vi "TP-PONDUL-INVERSE-PID.vi"() -> ()   [LabVIEW 2018]
uses:
  <vilib>/Instr/_visa.llb/VISA Configure Serial Port (Instr).vi
  <vilib>/addons/control/pid/pid.llb/PID (DBL).vi
  <vilib>/addons/control/pid/NI_PID_pid.lvlib
panel:
  in  "Tab Control":enum32{"Page 0", "Page 1", "Page 2"}(tab)
  out "Waveform Chart":dynamicdata(graph)
  in  "Consigne":dbl(knob) scale=-10.0..10.0
  out "Mesure":dbl(knob) scale=-50.0..50.0
  in  "stop":bool
  in  "VISA resource name":refnum<visa-resource-name>
  in  "PID gains":cluster{"P":dbl, "I":dbl, "D":dbl}={"P"=1.0, "I"=0.01, "D"=0.0} {"D" scale=0.0..28.0; "I" scale=0.0..0.0001; "P" scale=0.0..45.0}
  out "SPEED":dbl
  # "UNIVESITE SULTAN MOULAY SLIMANE\nFACULTE DES SCIENCES ET TECHNIQUES DE BENI MELLAL"
  # "Réalisé par : BANANE Mohamed\n               IDRRISI Hamza\n                      BELAISSAOUI ARBI\n                          TACHTIOUINE Hicham\n              CHAMIT Salim"
  # "Encadré par : Pr. KHAOUCH Zakaria"
  # "Placez tout \nd'abord le \npendule dans \nsa position d'equilibre \nverticale !"
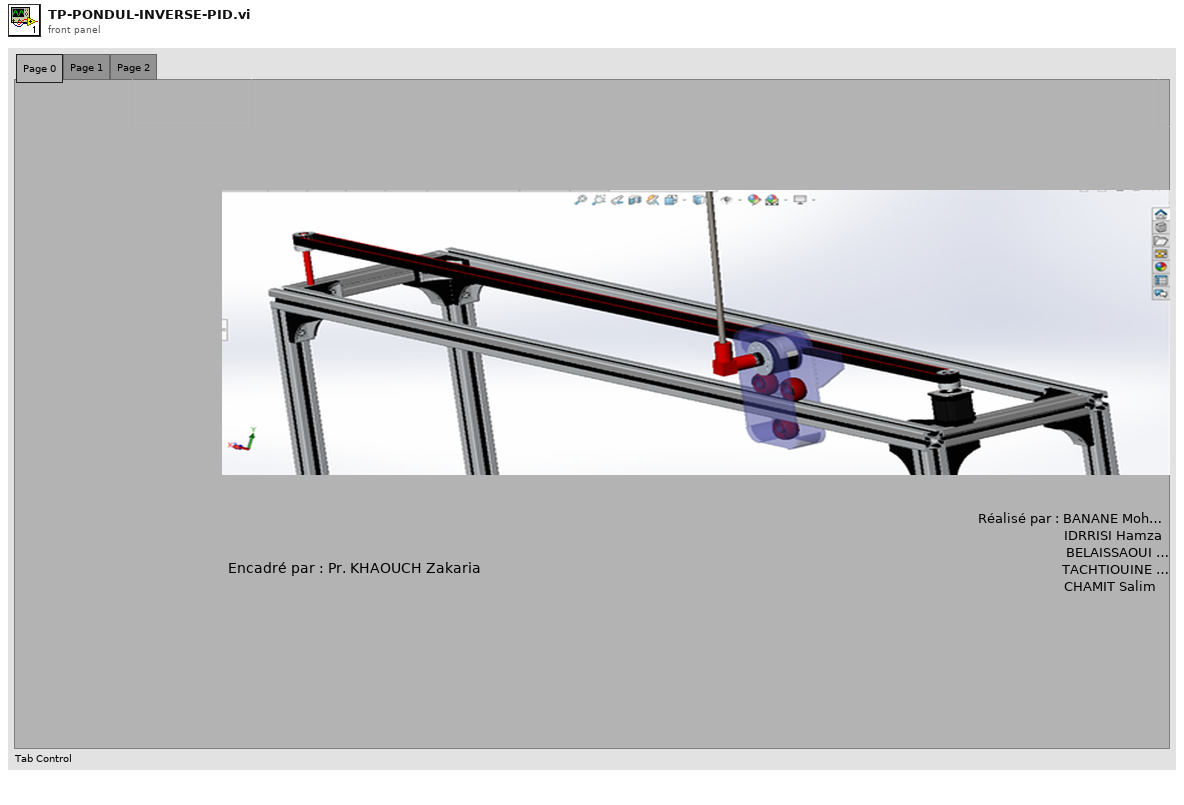
[diagram p1: front panel]
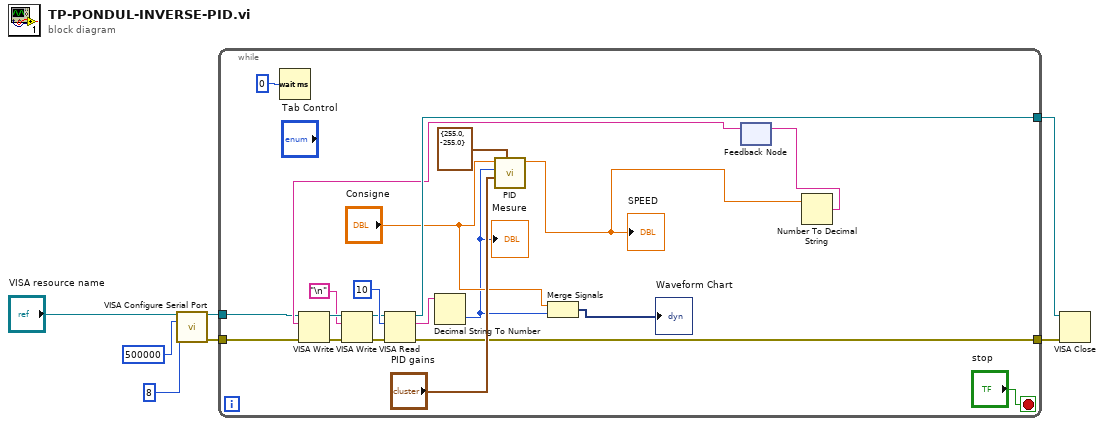
[diagram p0: block diagram]
diagram:
  n1 = call-poly "VISA Configure Serial Port"("VISA resource name"="VISA resource name", "baud rate (9600)"=u32 500000, "data bits (8)"=u16 8) -> ("VISA resource name out"=w3:refnum<visa-resource-name>, "error out"=w2:errorcluster)  [unwired: 11 in]
  n2 = while {
    tunnel: [w23] -> w4
    tunnel: [w22] -> w5
    tunnel: w3 -> [w18]
    tunnel: w2 -> [w17]
    stop <- "stop" stop-if-true
    n3 = Wait (ms)(milliseconds to wait=u32 0) -> ()  [unwired: 1 out]
    n4 = feedback #1() -> (w20:string)  [unwired: 1 in]
    n5 = VISA Write(VISA resource name=w18, write buffer=w20, error in (no error)=w17) -> (VISA resource name out=w16:refnum<visa-resource-name>, error out=w14:errorcluster)  [unwired: 1 out]
    n6 = VISA Write(VISA resource name=w16, write buffer="\n", error in (no error)=w14) -> (VISA resource name out=w15:refnum<visa-resource-name>, error out=w13:errorcluster)  [unwired: 1 out]
    n7 = VISA Read(VISA resource name=w15, byte count=u32 10, error in (no error)=w13) -> (VISA resource name out=w23:refnum<visa-resource-name>, read buffer=w26:string, error out=w22:errorcluster)  [unwired: 1 out]
    n8 = Decimal String To Number(string=w26) -> (number=w9:i32)  [unwired: 2 in, 1 out]
    "Mesure" <- w9
    n9 = call-poly <vilib>:"PID.vi"("output range"=cluster{"output high":dbl, "output low":dbl} {"output high"=255.0, "output low"=-255.0}, "PID gains"="PID gains", "process variable"=w9, "setpoint"="Consigne") -> ("output"=w8:dbl)  [unwired: 6 in, 1 out]
    "SPEED" <- w8
    n10 = Merge Signals("Consigne", w9) -> (→"Waveform Chart":dynamicdata)
    n11 = Number To Decimal String(number=w8) -> (decimal integer string=w21:string)  [unwired: 1 in]
    n12 = feedback-in #1(w21) -> ()
  }
  n13 = VISA Close(VISA resource name=w4, error in (no error)=w5) -> ()  [unwired: 1 out]
